vi "Initialize.vi"() -> (14 "Fatal Error Out":T4, 15 "State Out":T1)   [LabVIEW 2021, in "FirstXNode .xnode"]
uses:
  FirstXNode .xnode
  <vilib>/XNodeSupport/XNodeErrorCluster.ctl
  State.ctl
  <vilib>/XNodeSupport/XNodeBounds.ctl
  <vilib>/XNodeSupport/XNodeInt.ctl
  <vilib>/XNodeSupport/NI_XNodeSupport.lvlib
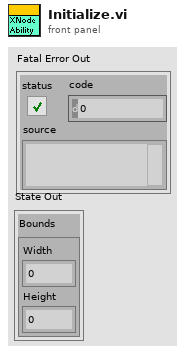
[diagram p1: front panel]
types:
  T1 = typedef "FirstXNode .xnode/State.ctl" = cluster{"Bounds":T2}
  T2 = typedef "NI_XNodeSupport.lvlib/XNodeBounds.ctl" = cluster{"Width":T3, "Height":T3}
  T3 = typedef "NI_XNodeSupport.lvlib/XNodeInt.ctl" = i32
  T4 = typedef "NI_XNodeSupport.lvlib/XNodeErrorCluster.ctl" = errorcluster
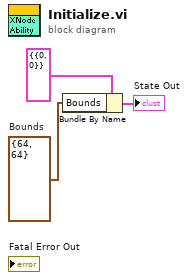
[diagram p0: block diagram]
diagram:
  w2 = T2 {"Width"=64, "Height"=64}  # Bounds
  n1 = Bundle By Name(cluster=T1 {"Bounds"={"Width"=0, "Height"=0}} ("State Out"), "Bounds"=w2) -> (→"State Out":T1)
